vi "RFmx_An_CHP_Disp.vi"(6 "CHP_Values":dbl[](array[numeric]) format="%#_6p", 9 "Int_Bandwidth":dbl, 10 "SignalBandwidth":dbl format="%#_6p", 11 "Input_Waveform":cluster{"x0":dbl, "dx":dbl, "y":sgl[]}) -> (3 "Waveform Graph 2":cluster{"x0":dbl, "dx":dbl, "y":sgl[]}[](graph))   [LabVIEW 2014]
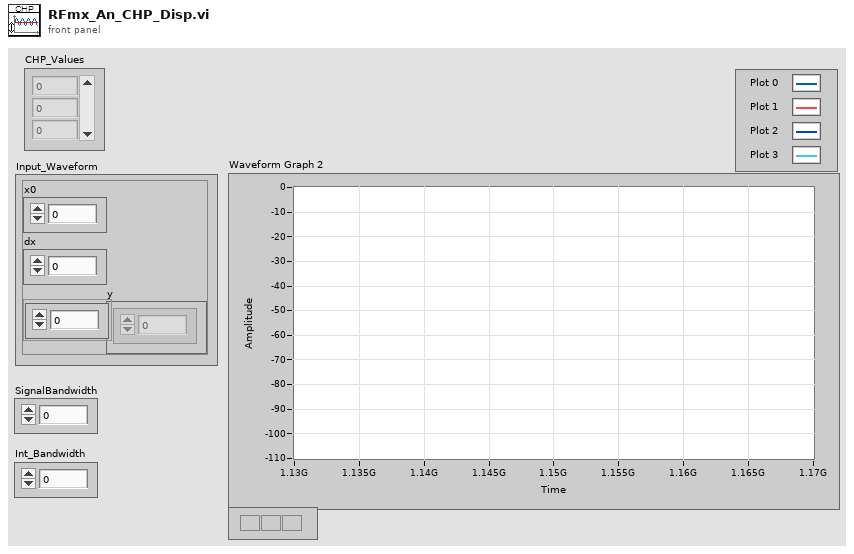
[diagram p1: front panel]
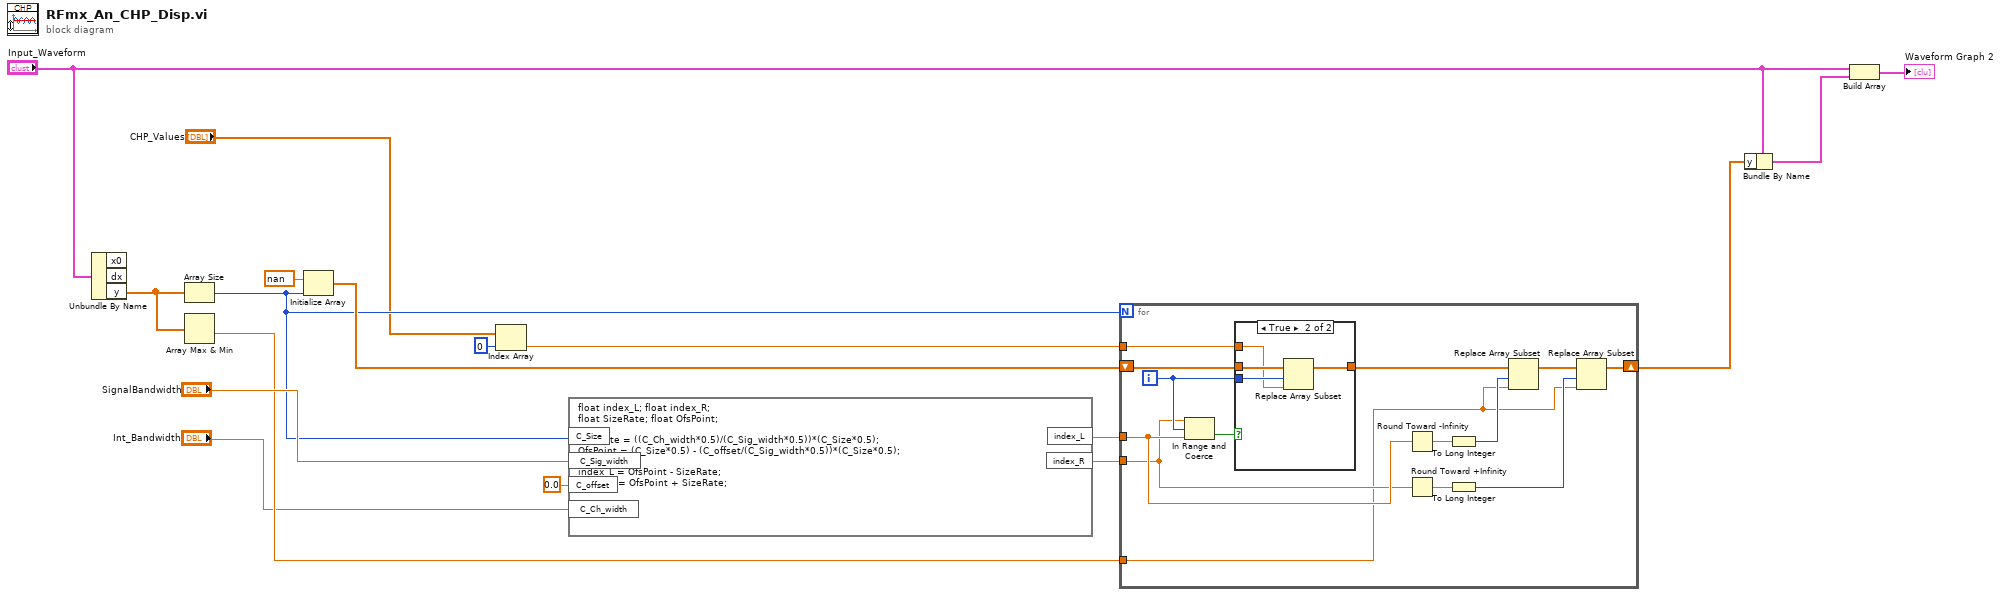
[diagram p0: block diagram]
diagram:
  n1 = Unbundle By Name("Input_Waveform") -> ("y"=w16:sgl[])  [unwired: 2 out]
  n2 = Array Size(array=w16) -> (size(s)=w10:i32)
  n3 = Array Max & Min(array=w16) -> (min value=w5:sgl)  [unwired: 3 out]
  n4 = Initialize Array(nan ("element"), w10) -> (w11:dbl[])
  n5 = Index Array(array="CHP_Values", index=0) -> (element=w1:dbl)
  n6 = formula code="float index_L; float index_R;\nfloat SizeRate; float OfsPoint;\n\nSizeRate = ((C_Ch_width*0.5)/(C_Sig_width*0.5))*(C_Size*0.5);\nOfsPoint = (C_Size*0.5) - (C_offset/(C_Sig_width*0.5))*(C_Size*0.5);\n\nindex_L = OfsPoint - SizeRate;\nindex_R = OfsPoint + SizeRate;"("C_Sig_width"="SignalBandwidth", "C_offset"=0.0 ("input variable"), "C_Ch_width"="Int_Bandwidth", "C_Size"=w10) -> ("index_L"=w8:dbl, "index_R"=w9:dbl)
  n7 = for {
    N: w10 -> [_]
    shift-right: [w19] -> w4
    shift-left: w11 -> [w31]
    tunnel: w9 -> [w21]
    tunnel: w8 -> [w22]
    tunnel: w5 -> [w20]
    tunnel: w1 -> [w18]
    i -> [w29]
    n8 = In Range and Coerce(upper limit=w21, x=w29, lower limit=w22) -> (In Range?=w30:bool)  [unwired: 1 out]
    n9 = case shown="True" w30 {
      tunnel: w31 -> [w32 w36]
      tunnel: w29 -> [_ w35]
      tunnel: [w32 w34] -> w23
      tunnel: w18 -> [_ w33]
      frame False {
      }
      frame True {
        n10 = Replace Array Subset(array=w36, new element=w33, index=w35) -> (w34:dbl[])
      }
    }
    n11 = Round Toward -Infinity(1:w22) -> (0:w28:dbl)
    n12 = Round Toward +Infinity(x=w21) -> (ceil(x): smallest int >= x=w27:dbl)
    n13 = To Long Integer(number=w28) -> (32bit integer=w26:i32)
    n14 = To Long Integer(number=w27) -> (32bit integer=w24:i32)
    n15 = Replace Array Subset(array=w23, new element=w20, index=w26) -> (w25:dbl[])
    n16 = Replace Array Subset(array=w25, new element=w20, index=w24) -> (w19:dbl[])
  }
  n17 = Bundle By Name(cluster="Input_Waveform", "y"=w4) -> (w2:cluster{"x0":dbl, "dx":dbl, "y":sgl[]})
  n18 = Build Array("Input_Waveform", w2) -> (→"Waveform Graph 2":cluster{"x0":dbl, "dx":dbl, "y":sgl[]}[])
